vi "Workspace.UI.DisableState.Set.vi"(7 "Mode.Tool?":bool, 8 "error in (no error)":errorcluster, 10 "Enable?":bool=TRUE, 11 "UI.Refs":T1) -> (0 "error out":errorcluster, 3 "UI.Refs out":T1)   [LabVIEW 2023, in "J1939 Workspace Shared.lvlib"]
uses:
  J1939 Workspace Shared.lvlib
  Types/UI.Refs.ctl
  SubModules/CAN-Streaming-Support/Source/Addon/Addon Shared/Types/Type Filter.ctl
  SubModules/CAN-Streaming-Support/Source/Addon/Addon Shared/Types/Direction Filter.ctl
  SubModules/CAN-Streaming-Support/Source/Addon/Addon Shared/CAN Stream Support Shared.lvlib
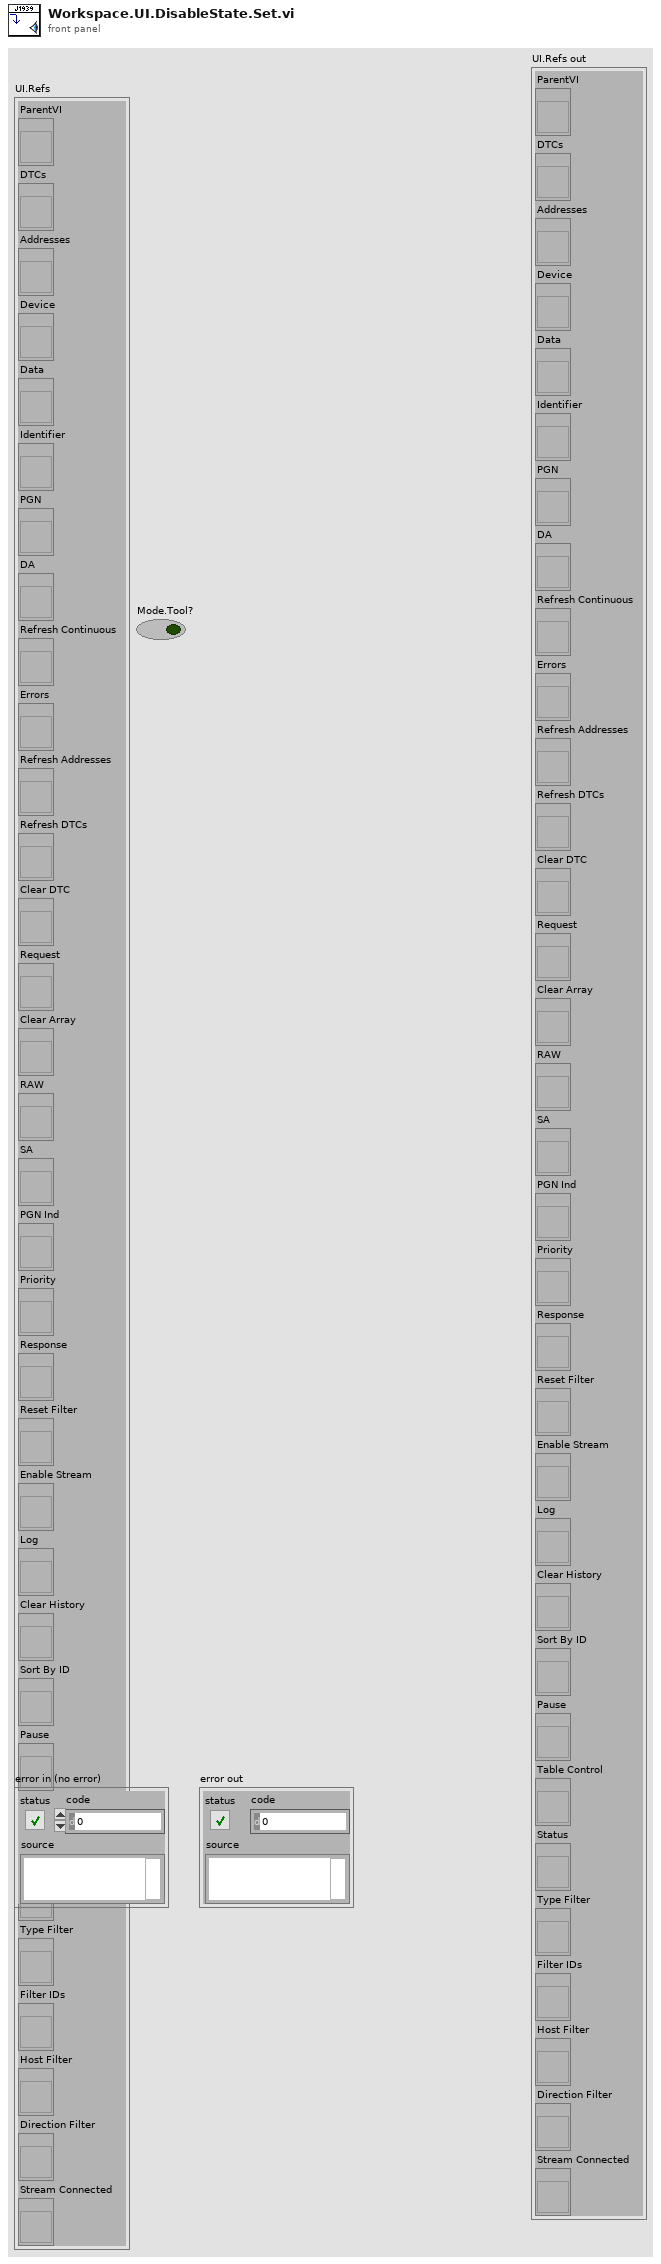
[diagram p1: front panel]
types:
  T1 = typedef "J1939 Workspace Shared.lvlib/UI.Refs.ctl" = cluster{"ParentVI":refnum<vi>, "DTCs":refnum<vi>, "Addresses":refnum<vi>, "Device":refnum<vi>, "Data":refnum<vi>, "Identifier":refnum<vi>, "PGN":refnum<vi>, "DA":refnum<vi>, "Refresh Continuous":refnum<vi>, "Errors":refnum<vi>, "Refresh Addresses":refnum<vi>, "Refresh DTCs":refnum<vi>, "Clear DTC":refnum<vi>, "Request":refnum<vi>, "Clear Array":refnum<vi>, "RAW":refnum<vi>, "SA":refnum<vi>, "PGN Ind":refnum<vi>, "Priority":refnum<vi>, "Response":refnum<vi>, "Reset Filter":refnum<vi>, "Enable Stream":refnum<vi>, "Log":refnum<vi>, "Clear History":refnum<vi>, "Sort By ID":refnum<vi>, "Pause":refnum<vi>, "Table Control":refnum<vi>, "Status":refnum<vi>, "Type Filter":refnum<vi>, "Filter IDs":refnum<vi>, "Host Filter":refnum<vi>, "Direction Filter":refnum<vi>, "Stream Connected":refnum<vi>}
  T2 = enum8{"Enabled", "Disabled", "Disabled and Grayed Out"}
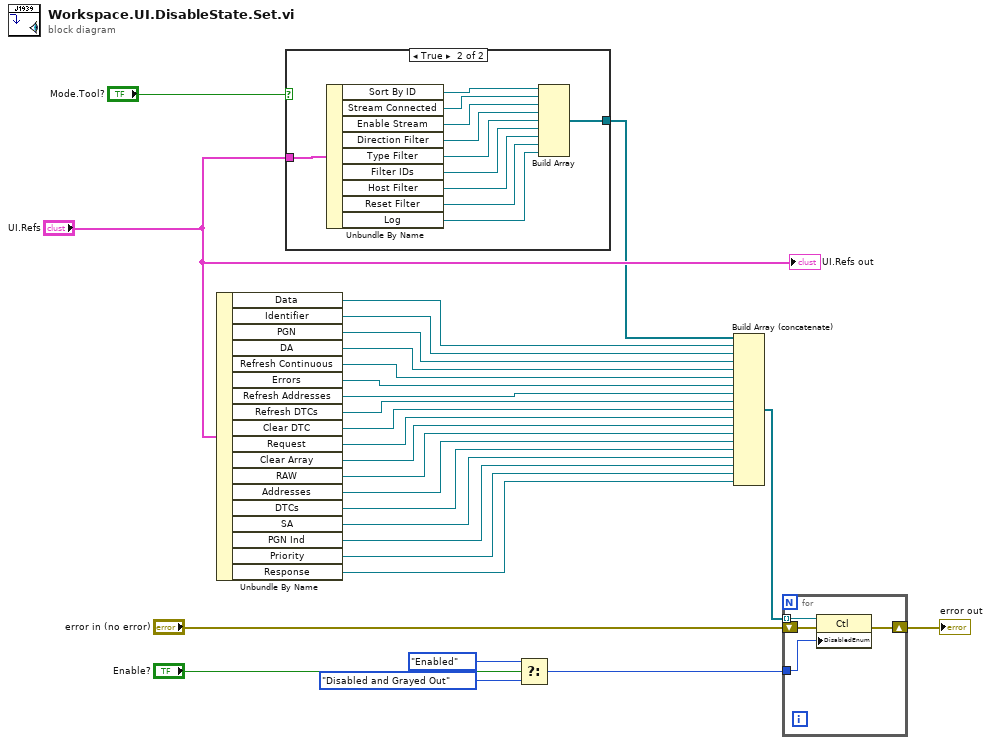
[diagram p0: block diagram]
diagram:
  n1 = Unbundle By Name("UI.Refs") -> ("Data"=w8:refnum<vi>, "Identifier"=w9:refnum<vi>, "PGN"=w10:refnum<vi>, "DA"=w11:refnum<vi>, "Refresh Continuous"=w12:refnum<vi>, "Errors"=w13:refnum<vi>, "Refresh Addresses"=w14:refnum<vi>, "Refresh DTCs"=w15:refnum<vi>, "Clear DTC"=w16:refnum<vi>, "Request"=w17:refnum<vi>, "Clear Array"=w18:refnum<vi>, "RAW"=w19:refnum<vi>, "Addresses"=w23:refnum<vi>, "DTCs"=w24:refnum<vi>, "SA"=w7:refnum<vi>, "PGN Ind"=w6:refnum<vi>, "Priority"=w5:refnum<vi>, "Response"=w4:refnum<vi>)
  n2 = case shown="True" "Mode.Tool?" {
    tunnel: "UI.Refs" -> [_ w30]
    tunnel: [_ w29] -> w2
    frame False {
    }
    frame True {
      n3 = Unbundle By Name(w30) -> ("Sort By ID"=w39:refnum<vi>, "Stream Connected"=w38:refnum<vi>, "Enable Stream"=w37:refnum<vi>, "Direction Filter"=w36:refnum<vi>, "Type Filter"=w35:refnum<vi>, "Filter IDs"=w34:refnum<vi>, "Host Filter"=w33:refnum<vi>, "Reset Filter"=w32:refnum<vi>, "Log"=w31:refnum<vi>)
      n4 = Build Array(w39, w38, w37, w36, w35, w34, w33, w32, w31) -> (w29:refnum<vi>[])
    }
  }
  n5 = Select(t=T2."Enabled" ("Disabled"), s="Enable?", f=T2."Disabled and Grayed Out" ("Disabled")) -> (s? t:f=w28:T2)
  n6 = Build Array (concatenate)(w2, w8, w9, w10, w11, w12, w13, w14, w15, w16, w17, w18, w19, w23, w24, w7, w6, w5, w4) -> (w21:refnum<vi>[])
  n7 = for {
    shift-right: [w41] -> w22
    shift-left: "error in (no error)" -> [w43]
    tunnel: w21 -> [w42] mode=indexing
    tunnel: w28 -> [w40]
    n8 = property class="Ctl"(reference=w42, error in=w43, "DisabledEnum"=w40) -> (error out=w41:errorcluster)  [unwired: 1 out]
  }
  "error out" <- w22
  "UI.Refs out" <- "UI.Refs"
